vi "SVL Exp Avg Sound Level.vi"   [LabVIEW 2017, in "SoundVib_SoundLevel.lvlib"]
doc: "Computes the exponential averaged sound level of <B>scaled signal [EU]</B>. <B>scaled signal [EU]</B> should have a zero DC component. Wire data to the <B>scaled signal [EU]</B> input to determine the polymorphic instance to use or manually select the instance."
uses:
  <vilib>/addons/Sound and Vibration/svt_Level/SoundVib_SoundLevel.lvlib
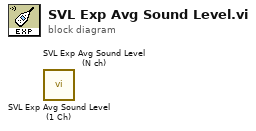
[diagram p0: block diagram]
diagram:
  n1 = call <vilib>:"SVL Exp Avg Sound Level (1 Ch).vi"() -> ()  [unwired: 7 in, 5 out]
  n2 = call <vilib>:"SVL Exp Avg Sound Level (N ch).vi"() -> ()  [unwired: 7 in, 5 out]
